vi "SCI_Rx_Access_0xB0.vi"(5 "串口读数据包（簇）":T1={"包头"=170, "数据低8位"=0, "数据低高8位"=0, "数据类型"=0, "CRC余数"=0, "数据无效"=FALSE, "数据更新"=FALSE} {"包头" format="%02x"; "数据低8位" format="%02x"; "数据低高8位" format="%02x"; "数据类型" items=["VOID"]; "CRC余数" format="%02x"}) -> (6 "包头":u16 format="%x", 8 "数据输出":u16 format="%x", 10 "CRC余数":u16 format="%x")   [LabVIEW 2015]
uses:
  SCI_DataPck.ctl
  SCI_DataType.ctl
panel:
  out "串口读数据包":T1={"包头"=170, "数据低8位"=0, "数据低高8位"=0, "数据类型"=0, "CRC余数"=0, "数据无效"=FALSE, "数据更新"=FALSE} {"包头" format="%02x"; "数据低8位" format="%02x"; "数据低高8位" format="%02x"; "数据类型" items=["VOID"]; "CRC余数" format="%02x"}
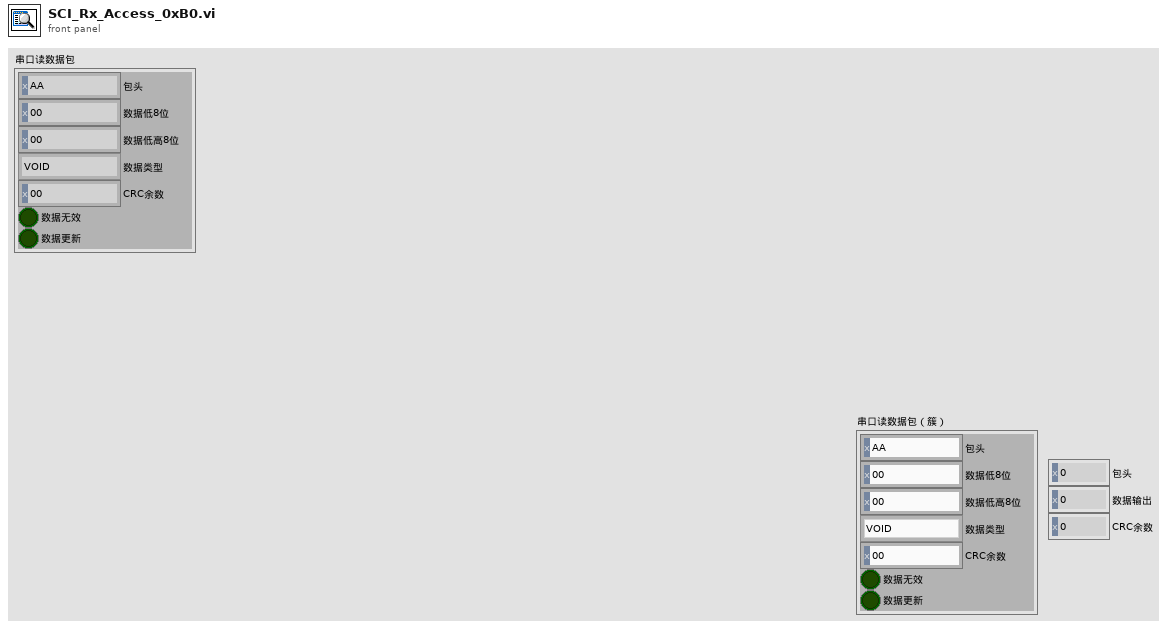
[diagram p1: front panel]
types:
  T1 = typedef "SCI_DataPck.ctl" = cluster{"包头":u16, "数据低8位":u16, "数据低高8位":u16, "数据类型":T2, "CRC余数":u16, "数据无效":bool, "数据更新":bool}
  T2 = typedef "SCI_DataType.ctl" = u16
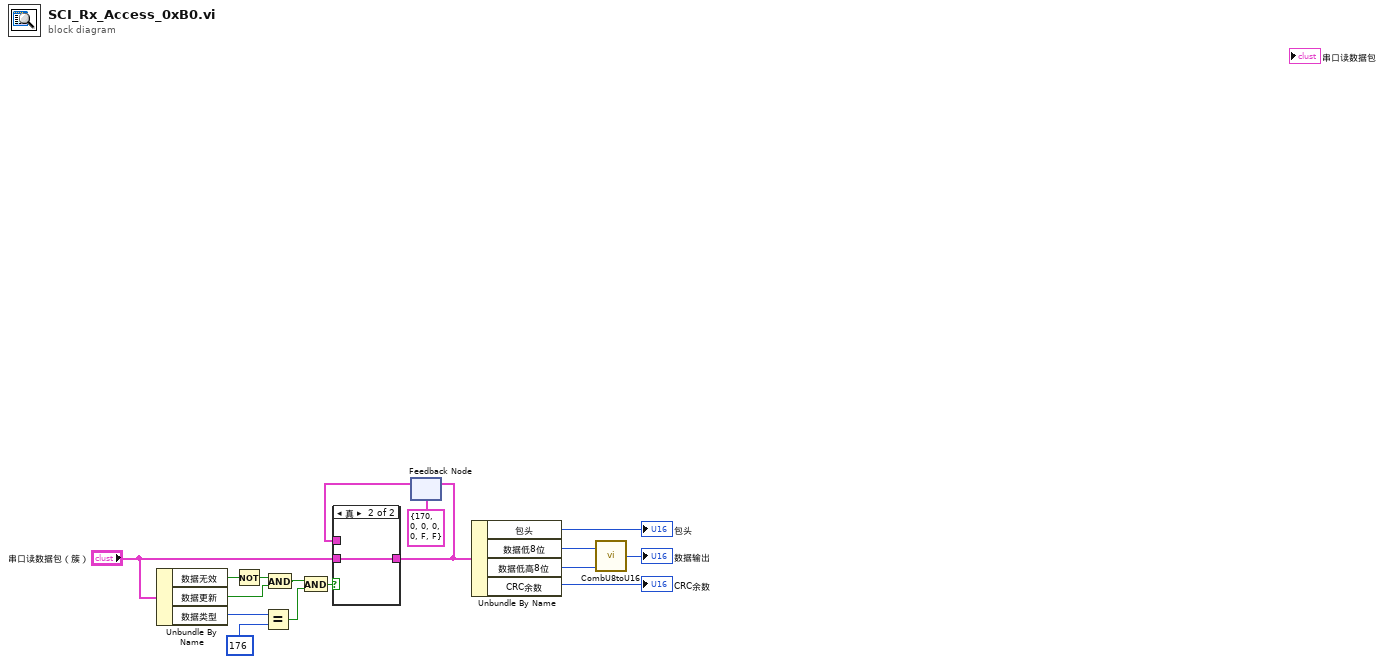
[diagram p0: block diagram]
diagram:
  n1 = Unbundle By Name("串口读数据包（簇）") -> ("数据无效"=w12:bool, "数据更新"=w11:bool, "数据类型"=w2:T2)
  n2 = Not(x=w12) -> (.not. x?=w16:bool)
  n3 = Equal?(x=w2, y=u16 176 ("数据类型")) -> (x = y?=w14:bool)
  n4 = And(x=w16, y=w11) -> (x .and. y?=w15:bool)
  n5 = And(x=w15, y=w14) -> (x .and. y?=w13:bool)
  n6 = feedback #1(T1 {"包头"=170, "数据低8位"=0, "数据低高8位"=0, "数据类型"=0, "CRC余数"=0, "数据无效"=FALSE, "数据更新"=FALSE} ("串口读簇")) -> (w10:T1)
  n7 = case shown="真" w13 {
    tunnel: [w18 w19] -> w3
    tunnel: "串口读数据包（簇）" -> [_ w19]
    tunnel: w10 -> [w18 _]
    frame False {
    }
    frame True {
    }
  }
  n8 = feedback-in #1(w3) -> ()
  n9 = Unbundle By Name(w3) -> ("包头"=→"包头":u16, "数据低8位"=w7:u16, "数据低高8位"=w6:u16, "CRC余数"=→"CRC余数":u16)
  n10 = call "CombU8toU16.vi"("数据高8位"=w6, "数据低8位"=w7) -> ("16位数据输出"=→"数据输出":u16)
